vi "ADAMPacer.vi"(4 "Scan Period":dbl format="%.2f", 5 "Previous Scan Value":dbl format="%.2f", 6 "Present scan array":dbl[](array[numeric]) format="%.2f", 7 "Value to Output":dbl format="%.2f", 8 "Ch Description":T1={"Ch Name"="", "Type"="", "Function"=enum."Analogue Input", "Ch State"=enum."On", "Calibration type"=enum."Raw", "A"=0.0, "B"=0.0, "C"=0.0, "D"=0.0, "Comments"="", "Address"={"Main"=0, "Ch."=0, "Sub"=0, "Port Name"=""}, "String"="", "Duty"=65535} {"Duty" format="%.0b"; "D" format="%#_5g"; "C" format="%#_5g"; "B" format="%#_5g"; "A" format="%#_5g"}, 9 "Ch names":string[](array[string])) -> (0 "Scan comment":string, 1 "Output":dbl format="%.3f", 3 "HelpText":string="\"A\" Warn if above this value\n\"B\" Warn if below this value\n\"C\" Hysteresis margin\n\"D\" is the averaging time in minutes\n\nWrite Channel name to check in the box above \"Comparator\"")   [LabVIEW 2015]
uses:
  ADAM Client/Sub VIs/ADAM Controls/Ch_description_ADAM.ctl
  ADAM Client/Sub VIs/ADAM Controls/Module_type_ADAM.ctl
  ADAM Client/Sub VIs/ADAM Controls/Function_ADAM.ctl
  ADAM Client/Sub VIs/ADAM Controls/Channel_State.ctl
  ADAM Client/Sub VIs/ADAM Controls/Calib_type_ADAM.ctl
  ADAM Client/Sub VIs/ADAM Controls/Address.ctl
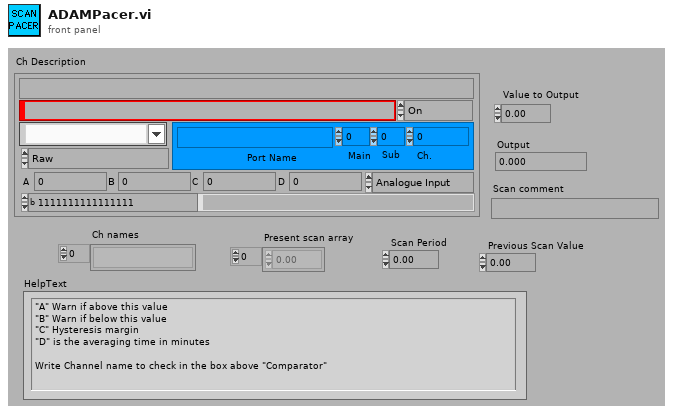
[diagram p1: front panel]
types:
  T1 = typedef "Ch_description_ADAM.ctl" = cluster{"Ch Name":string, "Type":T2, "Function":T3, "Ch State":T4, "Calibration type":T5, "A":dbl, "B":dbl, "C":dbl, "D":dbl, "Comments":string, "Address":T6, "String":string, "Duty":u16}
  T2 = typedef "Module_type_ADAM.ctl" = string
  T3 = typedef "Function_ADAM.ctl" = enum16{"Analogue Input", "Digital Input", "Event counter", "Event rate", "Analogue Output", "Digital Output", "Relay Output"}
  T4 = typedef "Channel_State.ctl" = enum16{"On", "Off", "Always On", "Always Off"}
  T5 = typedef "Calib_type_ADAM.ctl" = enum16{"Raw", "Bx + A", "Cx^2 + Bx + A", "Dx^3 + Cx^2 + Bx + A", "In Band", "Hi-Tec Q", "Hi-Tec M_dot", "Text"}
  T6 = typedef "Address.ctl" = cluster{"Main":i32, "Ch.":i32, "Sub":i32, "Port Name":string}
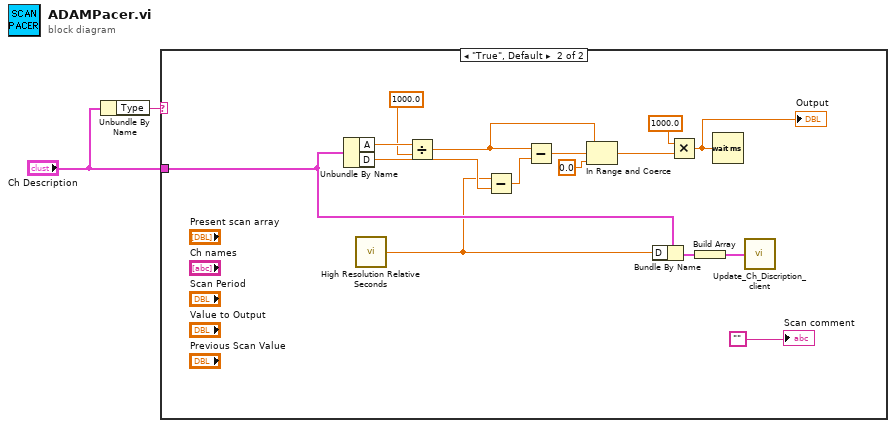
[diagram p0: block diagram]
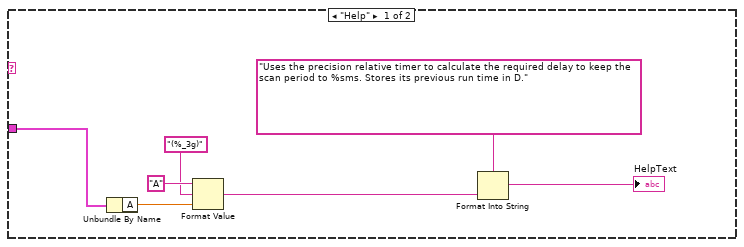
[diagram p2: hidden frame]
diagram:
  n1 = Unbundle By Name("Ch Description") -> ("Type"=w2:T2)
  n2 = case shown="\"True\", Default" w2 {
    tunnel: "Ch Description" -> [w6 w18]
    frame "Help" {
      n3 = Unbundle By Name(w6) -> ("A"=w8:dbl)
      n4 = Format Value(string ("")="A", format string="(%_3g)", value (0)=w8) -> (output string=w4:string)
      n5 = Format Into String(format string="Uses the precision relative timer to calculate the required delay to keep the scan period to %sms. Stores its previous run time in D.", w4) -> (resulting string=→"HelpText":string)  [unwired: 2 in, 1 out]
    }
    frame "True", Default {
      n6 = Unbundle By Name(w18) -> ("A"=w12:dbl, "D"=w23:dbl)
      n7 = call <vilib>:"High Resolution Relative Seconds.vi"() -> ("relative seconds"=w17:dbl)
      n8 = Divide(x=w12, y=1000.0 ("x")) -> (x/y=w11:dbl)
      n9 = Subtract(x=w17, y=w23) -> (x-y=w22:dbl)
      n10 = Subtract(x=w11, y=w22) -> (x-y=w21:dbl)
      n11 = In Range and Coerce(upper limit=w11, x=w21, lower limit=0.0) -> (coerced(x)=w14:dbl)  [unwired: 1 out]
      n12 = Bundle By Name(cluster=w18, "D"=w17) -> (w16:T1)
      n13 = Multiply(x=1000.0, y=w14) -> (x*y=w19:dbl)
      "Output" <- w19
      n14 = Build Array(w16) -> (w15:T1[])
      n15 = Wait (ms)(milliseconds to wait=w19) -> ()  [unwired: 1 out]
      n16 = call "Update_Ch_Discription_client.vi"("Channels to update In"=w15) -> ()  [unwired: 1 out]
      "Scan comment" <- ""
    }
  }
